vi "运维调试_氨氮.vi"() -> ()   [LabVIEW 2016, in "斯坦道氨氮.lvlib"]
uses:
  <vilib>/Utility/miscctls.llb/LVPointTypeDef.ctl
  <vilib>/Utility/config.llb/NI_LVConfig.lvlib
  <vilib>/ptbypt/NI_PtbyPt.lvlib
panel:
  in  "量程参数读取":T1
  in  "模块启用":bool
  in  "串口设置":bool
  in  "公式一键写入":bool
  in  "流程文件路径":path=path "C:/Users/STD/Documents/斯坦道流程文件/流程.xml"
  in  "曲线模型":cluster{"X^2":dbl, "X":dbl, "B":dbl}(xcontrol)
  in  "质控参数设置":bool
  out "字符串":string
  in  "氨氮自动测试量程配置":T2
  out "ADC":sgl
  out "温度2":sgl
  out "温度1":sgl
  out "固件版本号":string
  in  "数组":string[](array[string])
  in  "备用系数写入":bool
  in  "备用系数读取":bool
  in  "参数下拉列表":enum16{"氨氮", "总磷"}(ring)
  in  "量程下拉列表":enum16{"低量程", "高量程"}(ring)
  in  "测量模式下拉列表":enum16{"水样测量", "空白核查", "跨度核查", "标样核查", "加标回收"}(ring)
  in  "公式":cluster{"X^2":dbl, "X":dbl, "b":dbl}
  in  "写公式":bool
  in  "读公式":bool
  in  "返回":bool
  in  "设置":bool
  out "序列号":string="序列号"
  out "氨氮测量数据":T3(xcontrol)
  out "集成报警信息":string
  out "定时启动":bool
  out "总磷总氮运行状态":T4(xcontrol)
  in  "停止":bool
  in  "手动启动":bool
  in  "单步测试":bool
  in  "总磷氨氮调试":u16[](xcontrol)
  out "F3":sgl format="%#.6f"
  out "F2":sgl format="%#.6f"
  out "F1":sgl format="%#.6f"
  out "F0":sgl format="%#.6f"
  out "多列列表框":i32(listbox)
  # "参数设置"
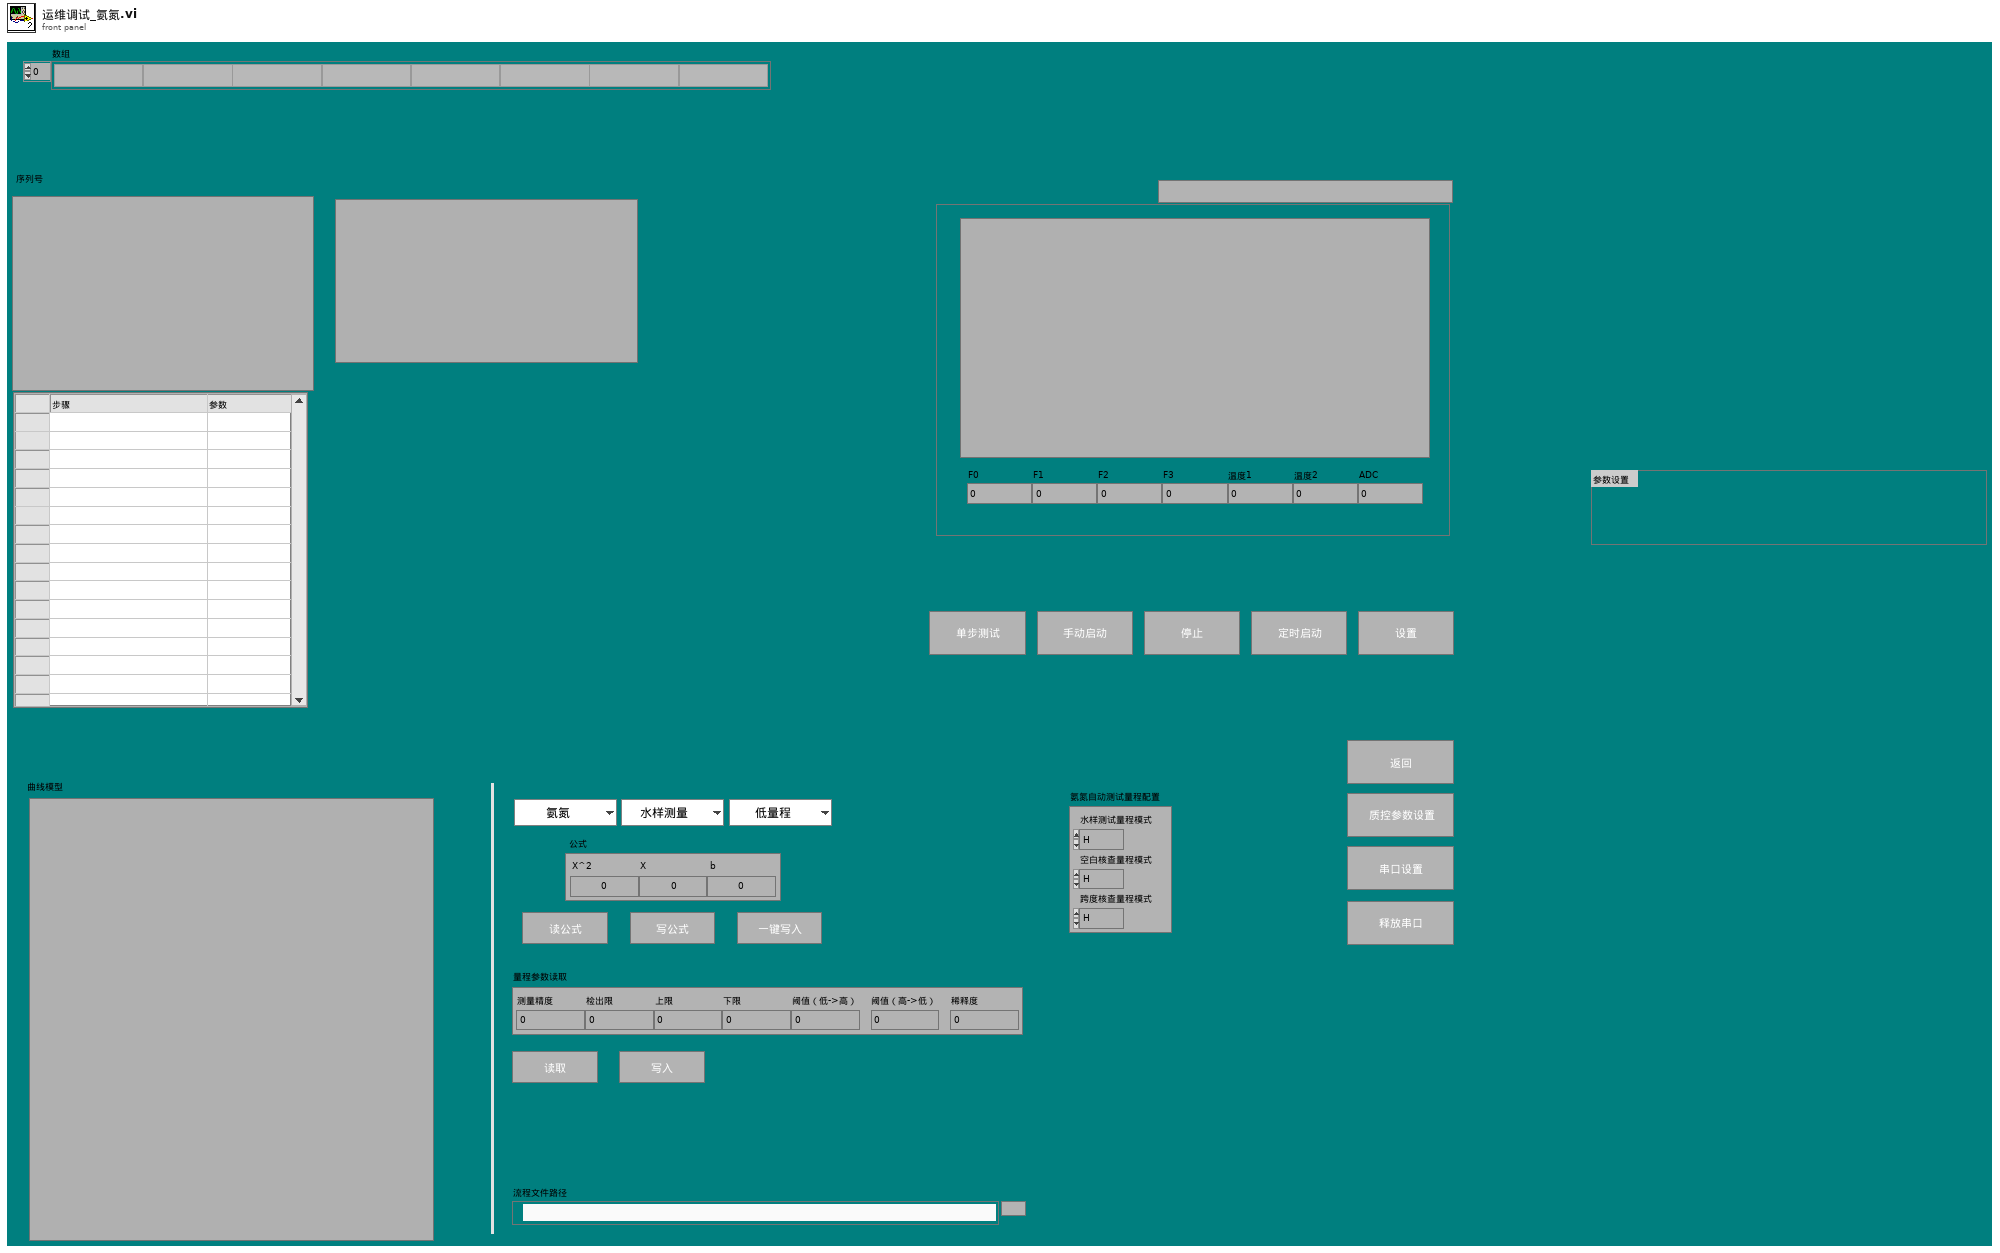
[diagram p1: front panel]
types:
  T1 = cluster{"测量精度":u16, "检出限":dbl, "上限":dbl, "下限":dbl, "阈值（低->高）":dbl, "阈值（高->低）":dbl, "稀释度":dbl}
  T2 = cluster{"水样测试量程模式":enum16{"H", "L", "AUTO"}, "空白核查量程模式":enum16{"H", "L", "AUTO"}, "跨度核查量程模式":enum16{"H", "L", "AUTO"}}
  T3 = cluster{"flowid":u16, "测量精度":u16, "测量数据区":cluster{"因子编码":u32, "单位":u16, "标样参考值":sgl, "水样数据时间":timestamp, "水样实测值":sgl, "水样数据标识":string, "标样数据时间":timestamp, "标样实测值":sgl, "标样数据标识":string, "空白数据时间":timestamp, "空白实测值":sgl, "空白数据标识":string, "零点核查数据时间":timestamp, "零点核查实测值":sgl, "零点核查数据标识":string, "跨度核查数据时间":timestamp, "跨度核查实测值":sgl, "跨度核查数据标识":string, "加标回收数据时间":timestamp, "加标回收实测值":sgl, "加标回收数据标识":string, "平行样数据时间":timestamp, "平行样实测值":sgl, "平行样数据标识":string, "F0":sgl, "F1":sgl, "F2":sgl, "F3":sgl, "F4":sgl, "F5":sgl, "F6":sgl, "F7":sgl, "温度":sgl, "湿度":sgl, "X值":sgl}}
  T4 = cluster{"系统时间":timestamp, "工作状态":enum16{"空闲", "水样测试", "标样核查", "零点核查", "跨度核查", "空白测试", "平行样测试", "加标回收", "空白校准", "标样校准", "初始化（清洗）"}, "测量模式":enum16{"待机", "连续模式", "周期模式", "定点模式", "受控模式", "手动模式"}, "告警代码":enum16{"无告警", "缺试剂告警", "缺水样告警", "缺蒸馏水告警", "缺标液告警", "仪表漏液告警", "标定异常告警", "超量程告警", "加热异常", "低试剂预警", "超上限告警", "超下限告警", "仪表内部其他异常", "滴定异常告警", "电极异常告警", "量程切换告警", "参数设置告警", "PH电极电位异常", "电导率电极异常", "浊度光度异常", "溶解氧电极异常", "溶解氧光强异常", "温度异常告警", "PH异常告警", "溶解氧异常告警", "电导率异常告警", "浊度异常告警", "叶绿素异常告警", "藻密度异常告警", "蓝绿藻异常告警", "ORP异常告警", "氨氮异常告警", "清洁刷异常告警", "SD卡异常告警", "蓝牙异常告警", "Wifi异常告警", "流程异常告警"}, "故障代码":enum16{"无故障", "电机故障", "温度故障", "通讯故障", "滴定故障"}, "日志代码":u16, "软件版本":u16, "F0":sgl, "F1":sgl, "F2":sgl, "F3":sgl, "T":sgl, "H":sgl, "id":u16, "flowid":u16, "量程":u16, "总磷控温温度1":sgl, "营养盐控温温度2":sgl, "ADC":sgl}
  T5 = enum16{"启动测量", "标样核查", "零点核查", "跨度核查", "空白测试", "平行样测试", "加标回收", "空白校准", "标样校准", "初始化（清洗）", "停止测试", "仪器重启", "校时", "模式设置", "测量间隔设置"}
  T6 = cluster{"仪器测试类型":enum16{"启动测量", "标样核查", "零点核查", "跨度核查", "空白测试", "平行样测试", "加标回收", "空白校准", "标样校准", "初始化（清洗）", "停止测试", "仪器重启", "校时", "模式设置", "测量间隔设置"}, "周期设置类型":enum16{"定点启动", "间隔启动"}, "定时功能启用":bool, "定时间隔":dbl, "24H周期设置":bool[], "空白核查时间":u16, "跨度核查时间":u16, "质控频次":enum16{"关闭", "每天", "星期一", "星期二", "星期三", "星期四", "星期五", "星期六", "星期日"}}
  T7 = enum16{"关闭", "每天", "星期一", "星期二", "星期三", "星期四", "星期五", "星期六", "星期日"}
  T8 = enum32{"Bad", "Idle", "Run top level", "Running"}
  T9 = typedef "LVDateTimeRec.ctl" = cluster{"秒数的小数部分":dbl, "秒":i32, "分":i32, "时":i32, "日":i32, "月":i32, "年":i32, "天数（周）":i32, "天数（年）":i32, "DST":i32}
  T10 = typedef "LVPointTypeDef.ctl" = cluster{"Horizontal":i16, "Vertical":i16}
  T11 = cluster{"因子编码":u32, "单位":u16, "标样参考值":sgl, "水样数据时间":timestamp, "水样实测值":sgl, "水样数据标识":string, "标样数据时间":timestamp, "标样实测值":sgl, "标样数据标识":string, "空白数据时间":timestamp, "空白实测值":sgl, "空白数据标识":string, "零点核查数据时间":timestamp, "零点核查实测值":sgl, "零点核查数据标识":string, "跨度核查数据时间":timestamp, "跨度核查实测值":sgl, "跨度核查数据标识":string, "加标回收数据时间":timestamp, "加标回收实测值":sgl, "加标回收数据标识":string, "平行样数据时间":timestamp, "平行样实测值":sgl, "平行样数据标识":string, "F0":sgl, "F1":sgl, "F2":sgl, "F3":sgl, "F4":sgl, "F5":sgl, "F6":sgl, "F7":sgl, "T":sgl, "H":sgl, "X":sgl}
  T12 = enum16{"空闲", "水样测试", "标样核查", "零点核查", "跨度核查", "空白测试", "平行样测试", "加标回收", "空白校准", "标样校准", "初始化（清洗）"}
  T13 = typedef "NI_LVConfig.lvlib/Config Data RefNum.ctl" = refnum<k1>
  T14 = cluster{"启动模式":enum16{"跨度核查", "水样测量", "空白核查", "标样核查", "加标回收"}, "启动参数":u16, "量程":enum16{"低量程", "高量程"}}
  T15 = cluster{"时间标识":timestamp, "设备":string, "日志信息":string, "流程参数":string}
  T16 = cluster{"时间标识":timestamp, "设备":string, "日志信息":string}
  T17 = enum16{"无告警", "缺试剂告警", "缺水样告警", "缺蒸馏水告警", "缺标液告警", "仪表漏液告警", "标定异常告警", "超量程告警", "加热异常", "低试剂预警", "超上限告警", "超下限告警", "仪表内部其他异常", "滴定异常告警", "电极异常告警", "量程切换告警", "参数设置告警", "PH电极电位异常", "电导率电极异常", "浊度光度异常", "溶解氧电极异常", "溶解氧光强异常", "温度异常告警", "PH异常告警", "溶解氧异常告警", "电导率异常告警", "浊度异常告警", "叶绿素异常告警", "藻密度异常告警", "蓝绿藻异常告警", "ORP异常告警", "氨氮异常告警", "清洁刷异常告警", "SD卡异常告警", "蓝牙异常告警", "Wifi异常告警", "流程异常告警"}
  T18 = typedef "LVRowAndColumnUnsignedTypeDef.ctl" = cluster{"Row":u32, "Column":u32}
  T19 = cluster{"站号":u16, "量程切换":enum32{"H", "L", "AUTO"}, "控制命令":enum16{"启动测量", "标样核查", "零点核查", "跨度核查", "空白测试", "平行样测试", "加标回收", "空白校准", "标样校准", "初始化（清洗）", "停止测试", "仪器重启", "校时", "模式设置", "测量间隔设置"}, "模式设置":enum16{"待机", "连续模式", "周期模式", "定点模式", "受控模式", "手动模式"}, "测量间隔":u16}
  T20 = cluster{"跨度值":dbl, "零点标准液浓度":dbl, "跨度标准液浓度":dbl, "标准液标准浓度":dbl}
  T21 = cluster{"确定":bool, "跨度值":dbl, "零点标准液浓度":dbl, "跨度标准液浓度":dbl, "标准液标准浓度":dbl}
  T22 = cluster{"控制命令":enum16{"启动测量", "标样核查", "零点核查", "跨度核查", "空白测试", "平行样测试", "加标回收", "空白校准", "标样校准", "初始化（清洗）", "停止测试", "仪器重启", "校时", "模式设置", "测量间隔设置"}, "周期设置类型":enum16{"定点启动", "间隔启动"}, "定时功能启用":bool, "定时间隔":dbl, "24H周期设置":bool[], "空白核查时间":u16, "跨度核查时间":u16, "质控频次":enum16{"关闭", "每天", "星期一", "星期二", "星期三", "星期四", "星期五", "星期六", "星期日"}}
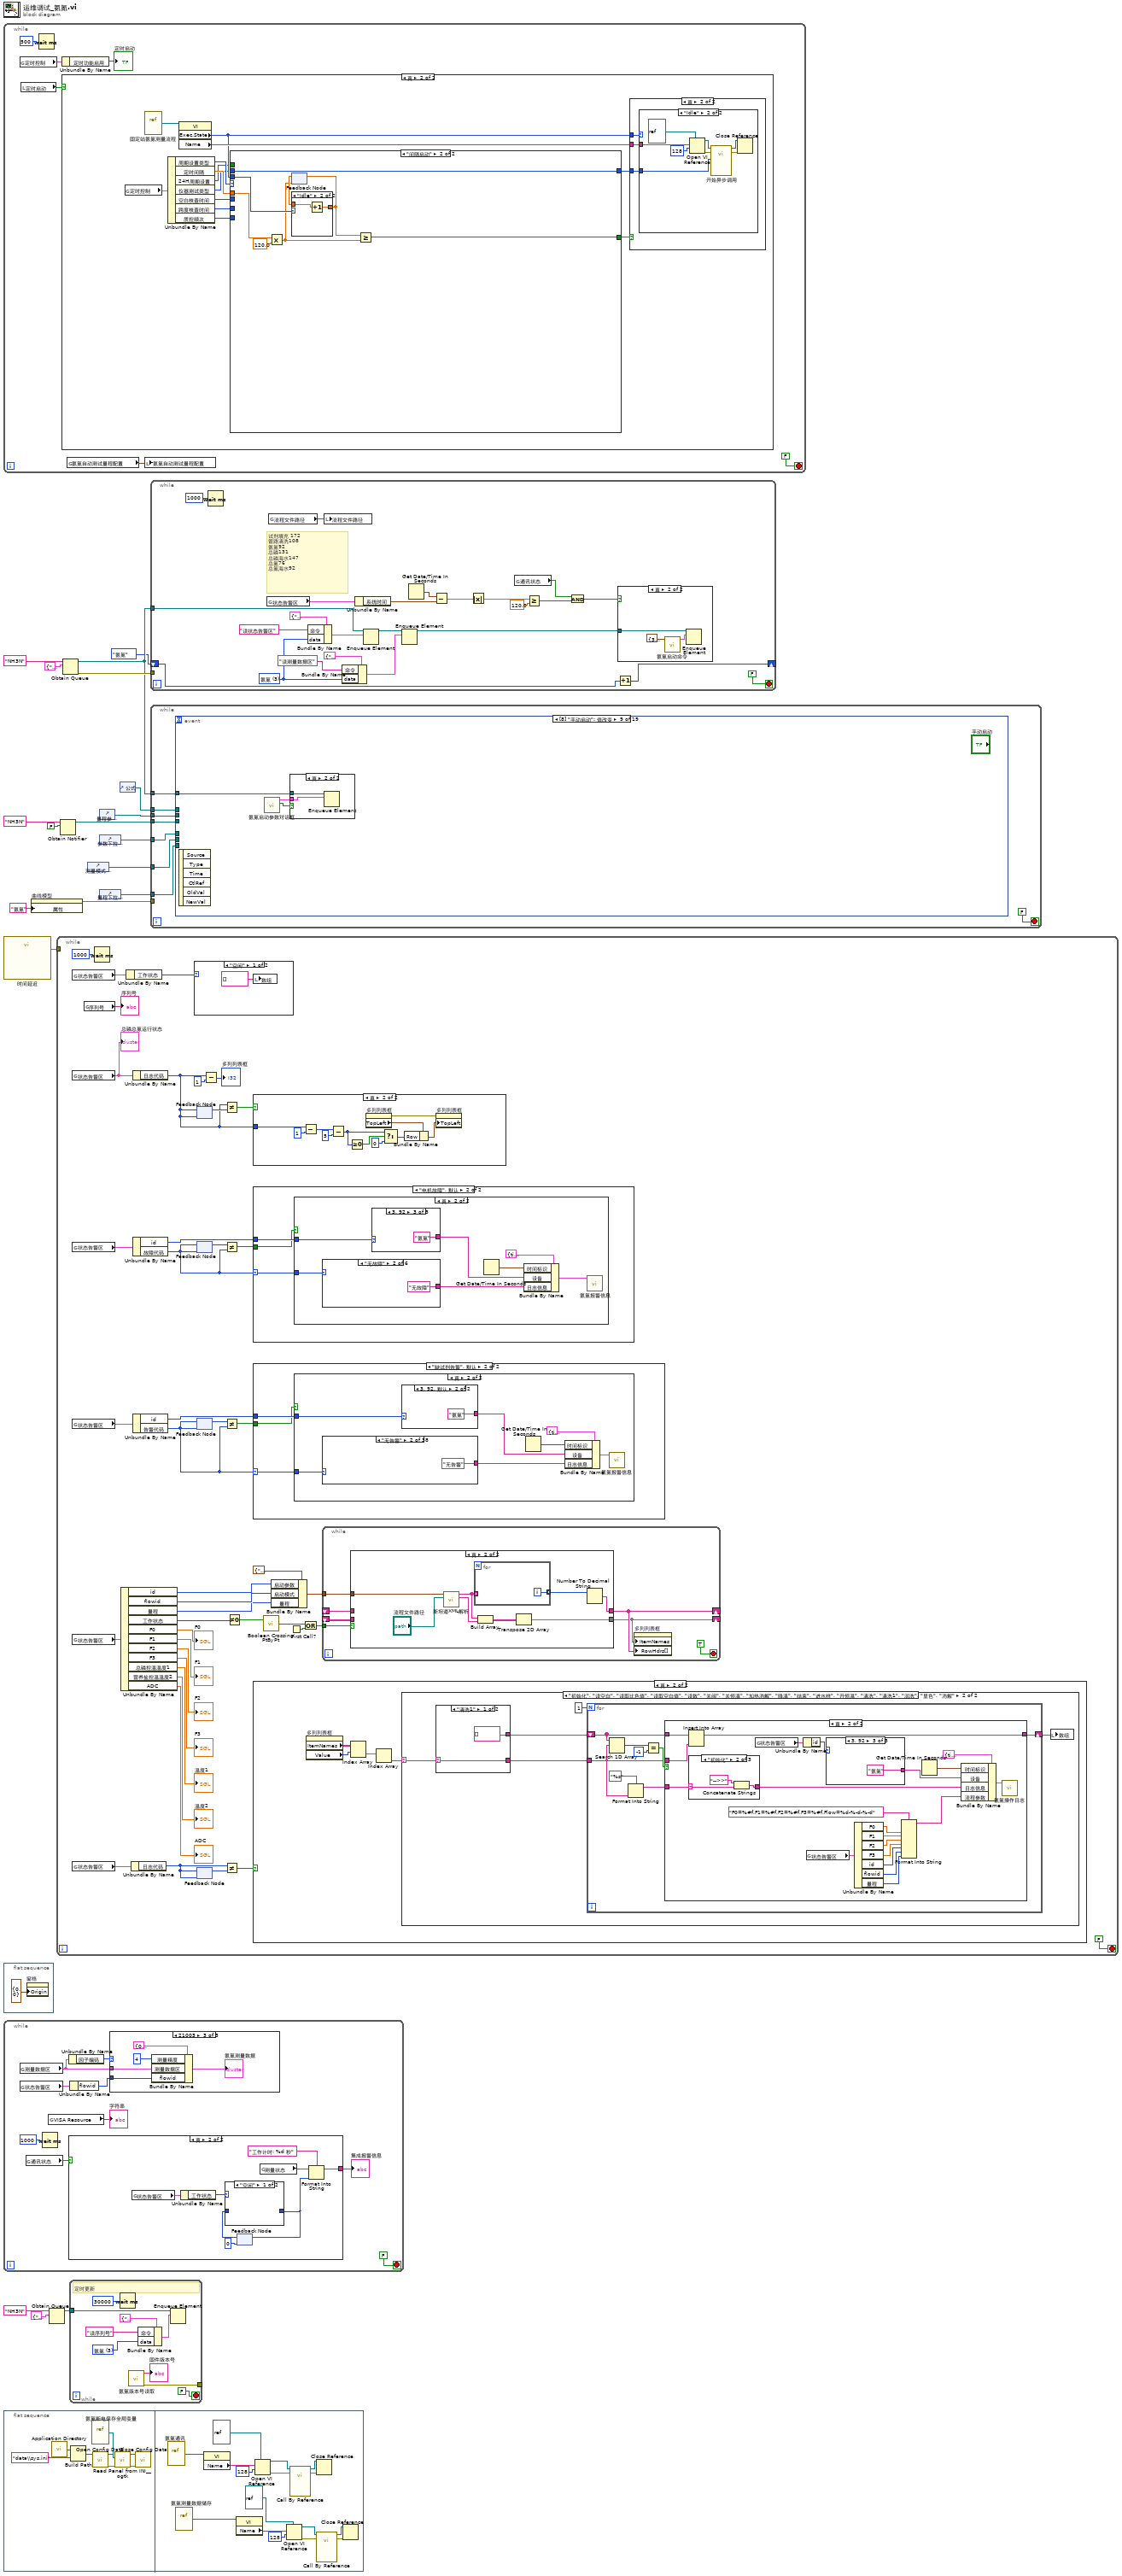
[diagram p0: block diagram]
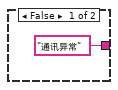
[diagram p2: hidden frame]
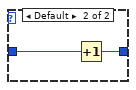
[diagram p3: hidden frame]
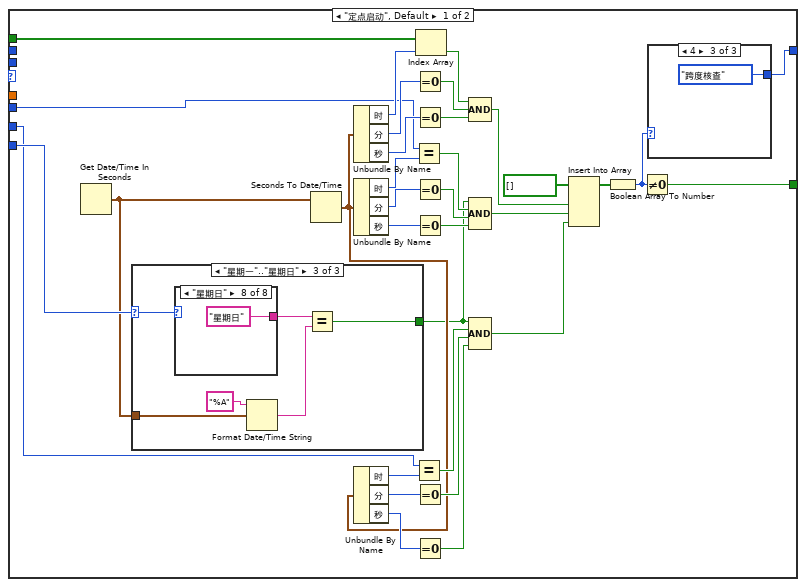
[diagram p7: hidden frame]
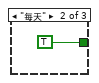
[diagram p9: hidden frame]
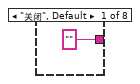
[diagram p10: hidden frame]
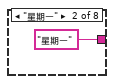
[diagram p11: hidden frame]
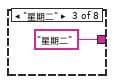
[diagram p12: hidden frame]
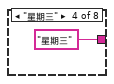
[diagram p13: hidden frame]
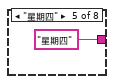
[diagram p14: hidden frame]
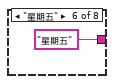
[diagram p15: hidden frame]
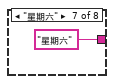
[diagram p16: hidden frame]
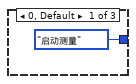
[diagram p17: hidden frame]
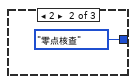
[diagram p18: hidden frame]
diagram:
  n1 = while {
    stop <- FALSE stop-if-true
    n2 = global read "氨氮断电保存全局变量.vi" "定时控制"() -> (w22:T6)
    n3 = local read "定时启动"() -> (w23:bool)
    n4 = Wait (ms)(milliseconds to wait=u32 500 ("等待时间（毫秒）")) -> ()  [unwired: 1 out]
    n5 = Unbundle By Name(w22) -> ("定时功能启用"=→"定时启动":bool)
    n6 = case shown="真" w23 {
      frame False {
      }
      frame True {
        n7 = global read "氨氮断电保存全局变量.vi" "定时控制"() -> (w38:T6)
        n8 = vi-ref "固定站氨氮测量流程.vi"() -> (w37:refnum<vi>)
        n9 = Unbundle By Name(w38) -> ("周期设置类型"=w34:enum16{"定点启动", "间隔启动"}, "定时间隔"=w33:dbl, "24H周期设置"=w32:bool[], "仪器测试类型"=w31:T5, "空白核查时间"=w30:u16, "跨度核查时间"=w29:u16, "质控频次"=w28:T7)
        n10 = property class="VI"(reference=w37) -> ("Exec.State"=w35:T8, "Name"=w36:string)  [unwired: 1 in, 2 out]
        n11 = case shown="\"间隔启动\"" w34 {
          tunnel: w33 -> [_ w94]
          tunnel: w32 -> [w62 _]
          tunnel: w35 -> [_ w97]
          tunnel: [w40 w92] -> w26
          tunnel: w31 -> [_ w90]
          tunnel: [w66 w90] -> w27
          tunnel: w28 -> [w65 _]
          tunnel: w30 -> [w58 _]
          tunnel: w29 -> [w47 _]
          frame "定点启动", Default {
            n12 = Get Date/Time In Seconds() -> (seconds since 1Jan1904=w64:timestamp)
            n13 = case shown="\"星期一\"..\"星期日\"" w65 {
              selector: w65 -> [_ _ w76]
              tunnel: w64 -> [_ _ w77]
              tunnel: [_ TRUE w73] -> w46
              frame "关闭", Default {
              }
              frame "每天" {
              }
              frame "星期一".."星期日" {
                n14 = case shown="\"星期日\"" w76 {
                  tunnel: ["" ("时间格式字符串(%c)") "星期一" ("时间格式字符串(%c)") "星期二" ("时间格式字符串(%c)") "星期三" ("时间格式字符串(%c)") "星期四" ("时间格式字符串(%c)") "星期五" ("时间格式字符串(%c)") "星期六" ("时间格式字符串(%c)") "星期日" ("时间格式字符串(%c)")] -> w75
                  frame "关闭", Default {
                  }
                  frame "星期一" {
                  }
                  frame "星期二" {
                  }
                  frame "星期三" {
                  }
                  frame "星期四" {
                  }
                  frame "星期五" {
                  }
                  frame "星期六" {
                  }
                  frame "星期日" {
                  }
                }
                n15 = Format Date/Time String(time format string (%c)="%A" ("时间格式字符串(%c)"), seconds (now)=w77) -> (date/time string=w74:string)  [unwired: 1 in]
                n16 = Equal?(x=w75, y=w74) -> (x = y?=w73:bool)
              }
            }
            n17 = Seconds To Date/Time(time stamp (now)=w64) -> (date time rec=w48:T9)  [unwired: 1 in]
            n18 = Unbundle By Name(w48) -> ("时"=w71:i32, "分"=w69:i32, "秒"=w70:i32)
            n19 = Unbundle By Name(w48) -> ("时"=w59:i32, "分"=w61:i32, "秒"=w60:i32)
            n20 = Unbundle By Name(w48) -> ("时"=w51:i32, "分"=w49:i32, "秒"=w50:i32)
            n21 = Equal?(x=w58, y=w59) -> (x = y?=w57:bool)
            n22 = Equal?(x=w47, y=w51) -> (x = y?=w52:bool)
            n23 = Equal To 0?(x=w69) -> (x = 0?=w68:bool)
            n24 = Equal To 0?(x=w70) -> (x = 0?=w67:bool)
            n25 = Equal To 0?(x=w61) -> (x = 0?=w56:bool)
            n26 = Equal To 0?(x=w60) -> (x = 0?=w55:bool)
            n27 = Equal To 0?(x=w49) -> (x = 0?=w53:bool)
            n28 = Equal To 0?(x=w50) -> (x = 0?=w54:bool)
            n29 = Index Array(array=w62, index=w71) -> (element=w63:bool)
            n30 = Compound Arithmetic op=AND ("复合运算")(w63, w68, w67) -> (w44:bool)
            n31 = Compound Arithmetic op=AND ("复合运算")(w46, w57, w56, w55) -> (w43:bool)
            n32 = Compound Arithmetic op=AND ("复合运算")(w46, w52, w53, w54) -> (w42:bool)
            n33 = Insert Into Array(array=bool[] [], new element #1=w44, new element #2=w43, new element #3=w42) -> (w41:bool[])  [unwired: 1 in]
            n34 = Boolean Array To Number(Boolean array=w41) -> (number=w39:u32)
            n35 = Not Equal To 0?(x=w39) -> (x != 0?=w40:bool)
            n36 = case shown="4" w39 {
              tunnel: [T5."启动测量" ("控制命令") T5."零点核查" ("控制命令") T5."跨度核查" ("控制命令")] -> w66
              frame 0, Default {
              }
              frame 2 {
              }
              frame 4 {
              }
            }
          }
          frame "间隔启动" {
            n37 = Multiply(x=w94, y=120.0) -> (x*y=w91:dbl)
            n38 = feedback #1(w91) -> (w96:dbl)
            n39 = case shown="\"Idle\"" w97 {
              tunnel: w96 -> [_ w99]
              tunnel: [_ w98] -> w95
              frame "Bad", Default {
              }
              frame "Idle" {
                n40 = Increment(x=w99) -> (x+1=w98:dbl)
              }
            }
            n41 = feedback-in #1(w95) -> ()
            n42 = Greater Or Equal?(x=w95, y=w91) -> (x >= y?=w92:bool)
          }
        }
        n43 = case shown="真" w26 {
          tunnel: w36 -> [_ w102]
          tunnel: w27 -> [_ w101]
          tunnel: w35 -> [_ w100]
          frame False {
          }
          frame True {
            n44 = case shown="\"Idle\"" w100 {
              tunnel: w102 -> [_ w106]
              tunnel: w101 -> [_ w103]
              frame "Bad", Default {
              }
              frame "Idle" {
                n45 = Open VI Reference(type specifier VI Refnum (for type only)=refnum<vi> refnum, vi path=w106, options=128 ("选项")) -> (vi reference=w107:refnum<vi>, error out=w108:errorcluster)  [unwired: 3 in]
                n46 = call-by-ref "开始异步调用"(reference=w107, error in=w108, "控制命令"=w103) -> (reference out=w109:refnum<vi>, error out=w110:errorcluster)  [unwired: 11 in]
                n47 = Close Reference(reference=w109, error in (no error)=w110) -> ()  [unwired: 1 out]
              }
            }
          }
        }
      }
    }
    n48 = global read "氨氮断电保存全局变量.vi" "氨氮自动测试量程配置"() -> (w20:T2)
    n49 = local write "氨氮自动测试量程配置"(w20) -> ()
  }
  n50 = call "时间延迟"() -> ("error out"=w10:errorcluster)  [unwired: 11 in]
  n51 = flat-sequence {
    frame #0 {
      n52 = property on="窗格" class="Pane"("Origin"=T10 {"Horizontal"=0, "Vertical"=0} ("原点")) -> ()  [unwired: 2 in, 2 out]
    }
  }
  n53 = while {
    stop <- FALSE stop-if-true
    n54 = global read "VAR氨氮全局变量.vi" "测量数据区"() -> (w118:T11)
    n55 = global read "VAR氨氮全局变量.vi" "状态告警区"() -> (w114:T4)
    n56 = global read "VAR氨氮全局变量.vi" "通讯状态"() -> (w116:bool)
    n57 = Wait (ms)(milliseconds to wait=u32 1000 ("等待时间（毫秒）")) -> ()  [unwired: 1 out]
    n58 = global read "氨氮断电保存全局变量.vi" "VISA Resource"() -> (→"字符串":refnum<visa-resource-name>)
    n59 = Unbundle By Name(w118) -> ("因子编码"=w117:u32)
    n60 = case shown="真" w116 {
      tunnel: ["通讯异常" ("集成报警信息") w123] -> w115
      frame False {
      }
      frame True {
        n61 = global read "VAR氨氮全局变量.vi" "状态告警区"() -> (w129:T4)
        n62 = Unbundle By Name(w129) -> ("工作状态"=w128:T12)
        n63 = feedback #2(0) -> (w126:i32)
        n64 = case shown="\"空闲\"" w128 {
          tunnel: w126 -> [_ w131]
          tunnel: [_ w130] -> w124
          frame "空闲" {
          }
          frame Default {
            n65 = Increment(x=w131) -> (x+1=w130:i32)
          }
        }
        n66 = feedback-in #2(w124) -> ()
        n67 = global read "VAR氨氮全局变量.vi" "测量状态"() -> (w122:string)
        n68 = Format Into String(format string="工作计时: %d 秒" ("格式字符串"), initial string=w122, w124) -> (resulting string=w123:string)  [unwired: 1 in, 1 out]
      }
    }
    "集成报警信息" <- w115
    n69 = Unbundle By Name(w114) -> ("flowid"=w113:u16)
    n70 = case shown="21003" w117 {
      tunnel: w118 -> [_ _ w136]
      tunnel: w113 -> [_ _ w134]
      frame Default {
      }
      frame 21011 {
      }
      frame 21003 {
        n71 = Bundle By Name(cluster=T3 {"flowid"=0, "测量精度"=0, "测量数据区"={"因子编码"=0, "单位"=0, "标样参考值"=0.0, "水样数据时间"=timestamp(0 s since 1904-01-01), "水样实测值"=0.0, "水样数据标识"="", "标样数据时间"=timestamp(0 s since 1904-01-01), "标样实测值"=0.0, "标样数据标识"="", "空白数据时间"=timestamp(0 s since 1904-01-01), "空白实测值"=0.0, "空白数据标识"="", "零点核查数据时间"=timestamp(0 s since 1904-01-01), "零点核查实测值"=0.0, "零点核查数据标识"="", "跨度核查数据时间"=timestamp(0 s since 1904-01-01), "跨度核查实测值"=0.0, "跨度核查数据标识"="", "加标回收数据时间"=timestamp(0 s since 1904-01-01), "加标回收实测值"=0.0, "加标回收数据标识"="", "平行样数据时间"=timestamp(0 s since 1904-01-01), "平行样实测值"=0.0, "平行样数据标识"="", "F0"=0.0, "F1"=0.0, "F2"=0.0, "F3"=0.0, "F4"=0.0, "F5"=0.0, "F6"=0.0, "F7"=0.0, "温度"=0.0, "湿度"=0.0, "X值"=0.0}} ("氨氮测量数据"), "测量精度"=u16 4, "测量数据区"=w136, "flowid"=w134) -> (→"氨氮测量数据":T3)
      }
    }
  }
  n72 = flat-sequence {
    frame #0 {
      n73 = call <vilib>:"Application Directory.vi"() -> ("Application Directory"=w137:path)
      n74 = Build Path(base path=w137, name or relative path="data\\sys.ini" ("名称或相对路径")) -> (appended path=w139:path)
      n75 = vi-ref "氨氮断电保存全局变量.vi"() -> (w141:refnum<vi>)
      n76 = call <vilib>:"Open Config Data.vi"("configuration file path"=w139) -> ("error out"=w143:errorcluster, "refnum"=w140:T13)  [unwired: 8 in, 1 out]
      n77 = call <userlib>:"Read Panel from INI__ogtk.vi"("error in (no error)"=w143, "VI ref"=w141, "refnum"=w140) -> ("error out"=w144:errorcluster, "refnum out"=w142:T13)  [unwired: 7 in]
      n78 = call <vilib>:"Close Config Data.vi"("error in (no error)"=w144, "refnum"=w142) -> ()  [unwired: 8 in, 2 out]
    }
    frame #1 {
      n79 = vi-ref "氨氮通讯.vi"() -> (w160:refnum<vi>)
      n80 = vi-ref "氨氮测量数据储存.vi"() -> (w152:refnum<vi>)
      n81 = property class="VI"(reference=w160) -> ("Name"=w159:string)  [unwired: 1 in, 2 out]
      n82 = property class="VI"(reference=w152) -> ("Name"=w145:string)  [unwired: 1 in, 2 out]
      n83 = Open VI Reference(type specifier VI Refnum (for type only)=refnum<vi> refnum, vi path=w159, options=128 ("选项")) -> (vi reference=w157:refnum<vi>, error out=w155:errorcluster)  [unwired: 3 in]
      n84 = Open VI Reference(type specifier VI Refnum (for type only)=refnum<vi> refnum, vi path=w145, options=128 ("选项")) -> (vi reference=w147:refnum<vi>, error out=w149:errorcluster)  [unwired: 3 in]
      n85 = call-by-ref "?"(reference=w157, error in=w155) -> (reference out=w153:refnum<vi>, error out=w154:errorcluster)  [unwired: 12 in]
      n86 = Close Reference(reference=w153, error in (no error)=w154) -> ()  [unwired: 1 out]
      n87 = call-by-ref "?"(reference=w147, error in=w149) -> (reference out=w151:refnum<vi>, error out=w150:errorcluster)  [unwired: 12 in]
      n88 = Close Reference(reference=w151, error in (no error)=w150) -> ()  [unwired: 1 out]
    }
  }
  n89 = property on="曲线模型" class="曲线模型 (严格)"("属性"="氨氮" ("调用模块名称属性")) -> (error out=w3:errorcluster)  [unwired: 2 in, 1 out]
  n90 = Obtain Queue(name (unnamed)="NH3N" ("名称（未命名）"), element data type=cluster{"命令":string, "data":variant} {"命令"="", "data"=variant}) -> (queue out=w7:refnum<queue>)  [unwired: 3 in, 2 out]
  n91 = while {
    tunnel: w10 -> [_]
    stop <- FALSE stop-if-true
    n92 = global read "VAR氨氮全局变量.vi" "状态告警区"() -> (w176:T4)
    n93 = global read "VAR氨氮全局变量.vi" "状态告警区"() -> (w188:T4)
    "总磷总氮运行状态" <- w188
    n94 = global read "VAR氨氮全局变量.vi" "状态告警区"() -> (w181:T4)
    n95 = global read "VAR氨氮全局变量.vi" "状态告警区"() -> (w186:T4)
    n96 = global read "VAR氨氮全局变量.vi" "状态告警区"() -> (w196:T4)
    n97 = global read "VAR氨氮全局变量.vi" "状态告警区"() -> (w173:T4)
    n98 = global read "VAR氨氮全局变量.vi" "序列号"() -> (→"序列号":string)
    n99 = Wait (ms)(milliseconds to wait=u32 1000 ("等待时间（毫秒）")) -> ()  [unwired: 1 out]
    n100 = Unbundle By Name(w196) -> ("id"=w193:u16, "flowid"=w195:u16, "量程"=w194:u16, "工作状态"=w162:T12, "F0"=→"F0":sgl, "F1"=→"F1":sgl, "F2"=→"F2":sgl, "F3"=→"F3":sgl, "总磷控温温度1"=→"温度1":sgl, "营养盐控温温度2"=→"温度2":sgl, "ADC"=→"ADC":sgl)
    n101 = Unbundle By Name(w176) -> ("工作状态"=w175:T12)
    n102 = Unbundle By Name(w173) -> ("日志代码"=w172:u16)
    n103 = Unbundle By Name(w188) -> ("日志代码"=w166:u16)
    n104 = Unbundle By Name(w181) -> ("id"=w180:u16, "故障代码"=w177:enum16{"无故障", "电机故障", "温度故障", "通讯故障", "滴定故障"})
    n105 = Unbundle By Name(w186) -> ("id"=w185:u16, "告警代码"=w182:T17)
    n106 = case shown="\"空闲\"" w175 {
      frame "空闲" {
        n107 = local write "数组"(string[] [] ("数组")) -> ()
      }
      frame "水样测试", Default {
      }
    }
    n108 = feedback-in #3(w166) -> ()
    n109 = feedback #3(w166) -> (w201:u16)
    n110 = feedback #4(w177) -> (w178:enum16{"无故障", "电机故障", "温度故障", "通讯故障", "滴定故障"})
    n111 = feedback-in #4(w177) -> ()
    n112 = feedback #5(w182) -> (w183:T17)
    n113 = feedback-in #5(w182) -> ()
    n114 = feedback #6(w172) -> (w174:u16)
    n115 = feedback-in #6(w172) -> ()
    n116 = Subtract(x=w166, y=1) -> (x-y=→"多列列表框":i32)
    n117 = Not Equal?(x=w166, y=w201) -> (x != y?=w200:bool)
    n118 = Not Equal?(x=w178, y=w177) -> (x != y?=w179:bool)
    n119 = Not Equal?(x=w183, y=w182) -> (x != y?=w184:bool)
    n120 = Not Equal?(x=w172, y=w174) -> (x != y?=w171:bool)
    n121 = Not Equal To 0?(x=w162) -> (x != 0?=w198:bool)
    n122 = case shown="真" w200 {
      tunnel: w166 -> [_ w351]
      frame False {
      }
      frame True {
        n123 = Subtract(x=w351, y=1) -> (x-y=w349:i32)
        n124 = Subtract(x=w349, y=5) -> (x-y=w353:i32)
        n125 = Greater Or Equal To 0?(x=w353) -> (x >= 0?=w352:bool)
        n126 = property on="多列列表框" class="MCListbox (严格)"() -> (error out=w357:errorcluster, "TopLeft"=w358:T18)  [unwired: 2 in, 1 out]
        n127 = Select(t=w353, s=w352, f=0) -> (s? t:f=w354:i32)
        n128 = Bundle By Name(cluster=w358, "Row"=w354) -> (w359:T18)
        n129 = property on="多列列表框" class="MCListbox (严格)"(error in=w357, "TopLeft"=w359) -> ()  [unwired: 1 in, 2 out]
      }
    }
    n130 = case shown="\"电机故障\", 默认" w177 {
      selector: w177 -> [_ w258]
      tunnel: w180 -> [_ w259]
      tunnel: w179 -> [_ w257]
      frame "无故障" {
      }
      frame "电机故障", Default {
        n131 = case shown="真" w257 {
          tunnel: w259 -> [_ w266]
          tunnel: w258 -> [_ w261]
          frame False {
          }
          frame True {
            n132 = case shown="\"无故障\"" w261 {
              selector: w261 -> [w268 _ _ _ _ _]
              tunnel: [w267 "无故障" "电机故障" "温度故障" "通讯故障" "滴定故障"] -> w260
              frame Default {
                n133 = Format Into String(format string="%d" ("格式字符串"), initial string="未知" ("工作状态"), w268) -> (resulting string=w267:string)  [unwired: 1 in, 1 out]
              }
              frame "无故障" {
              }
              frame "电机故障" {
              }
              frame "温度故障" {
              }
              frame "通讯故障" {
              }
              frame "滴定故障" {
              }
            }
            n134 = case shown="3, 92" w266 {
              tunnel: [_ "总磷" ("table输入") "氨氮" ("table输入")] -> w262
              frame Default {
              }
              frame 1, 131 {
              }
              frame 3, 92 {
              }
            }
            n135 = Get Date/Time In Seconds() -> (seconds since 1Jan1904=w263:timestamp)
            n136 = Bundle By Name(cluster=T16 {"时间标识"=timestamp(0 s since 1904-01-01), "设备"="", "日志信息"=""} ("data in"), "时间标识"=w263, "设备"=w262, "日志信息"=w260) -> (w264:T16)
            n137 = call "氨氮报警信息.vi"("data in"=w264) -> ()  [unwired: 10 in, 1 out]
          }
        }
      }
    }
    n138 = case shown="\"缺试剂告警\", 默认" w182 {
      selector: w182 -> [_ w279]
      tunnel: w185 -> [_ w280]
      tunnel: w184 -> [_ w278]
      frame "无告警" {
      }
      frame "缺试剂告警", Default {
        n139 = case shown="真" w278 {
          tunnel: w280 -> [_ w287]
          tunnel: w279 -> [_ w281]
          frame False {
          }
          frame True {
            n140 = case shown="\"无告警\"" w281 {
              selector: w281 -> [w289 _ _ _ _ _ _ _ _ _ _ _ _ _ _ _ _ _ _ _ _ _ _ _ _ _ _ _ _ _ _ _ _ _ _ _ _ _]
              tunnel: [w288 "无告警" "缺试剂告警" "缺水样告警" "缺蒸馏水告警" "缺标液告警" "仪表漏液告警" "标定异常告警" "超量程告警" "加热异常" "低试剂预警" "超上限告警" "超下限告警" "仪表内部其他异常" "滴定异常告警" "电极异常告警" "量程切换告警" "参数设置告警" "PH电极电位异常" "电导率电极异常" "浊度光度异常" "溶解氧电极异常" "溶解氧光强异常" "温度异常告警" "PH异常告警" "溶解氧异常告警" "电导率异常告警" "浊度异常告警" "叶绿素异常告警" "藻密度异常告警" "蓝绿藻异常告警" "ORP异常告警" "氨氮异常告警" "清洁刷异常告警" "SD卡异常告警" "蓝牙异常告警" "WiFi异常告警" "流程异常告警"] -> w282
              frame Default {
                n141 = Format Into String(format string="%d" ("格式字符串"), initial string="未知" ("工作状态"), w289) -> (resulting string=w288:string)  [unwired: 1 in, 1 out]
              }
              frame "无告警" {
              }
              frame "缺试剂告警" {
              }
              frame "缺水样告警" {
              }
              frame "缺蒸馏水告警" {
              }
              frame "缺标液告警" {
              }
              frame "仪表漏液告警" {
              }
              frame "标定异常告警" {
              }
              frame "超量程告警" {
              }
              frame "加热异常" {
              }
              frame "低试剂预警" {
              }
              frame "超上限告警" {
              }
              frame "超下限告警" {
              }
              frame "仪表内部其他异常" {
              }
              frame "滴定异常告警" {
              }
              frame "电极异常告警" {
              }
              frame "量程切换告警" {
              }
              frame "参数设置告警" {
              }
              frame "PH电极电位异常" {
              }
              frame "电导率电极异常" {
              }
              frame "浊度光度异常" {
              }
              frame "溶解氧电极异常" {
              }
              frame "溶解氧光强异常" {
              }
              frame "温度异常告警" {
              }
              frame "PH异常告警" {
              }
              frame "溶解氧异常告警" {
              }
              frame "电导率异常告警" {
              }
              frame "浊度异常告警" {
              }
              frame "叶绿素异常告警" {
              }
              frame "藻密度异常告警" {
              }
              frame "蓝绿藻异常告警" {
              }
              frame "ORP异常告警" {
              }
              frame "氨氮异常告警" {
              }
              frame "清洁刷异常告警" {
              }
              frame "SD卡异常告警" {
              }
              frame "蓝牙异常告警" {
              }
              frame "Wifi异常告警" {
              }
              frame "流程异常告警" {
              }
            }
            n142 = case shown="3, 92, 默认" w287 {
              tunnel: ["总磷" ("table输入") "氨氮" ("table输入")] -> w283
              frame 1, 131 {
              }
              frame 3, 92, Default {
              }
            }
            n143 = Get Date/Time In Seconds() -> (seconds since 1Jan1904=w284:timestamp)
            n144 = Bundle By Name(cluster=T16 {"时间标识"=timestamp(0 s since 1904-01-01), "设备"="", "日志信息"=""} ("data in"), "时间标识"=w284, "设备"=w283, "日志信息"=w282) -> (w285:T16)
            n145 = call "氨氮报警信息.vi"("data in"=w285) -> ()  [unwired: 10 in, 1 out]
          }
        }
      }
    }
    n146 = case shown="真" w171 {
      frame False {
      }
      frame True {
        n147 = property on="多列列表框" class="MCListbox (严格)"() -> ("ItemNames"=w207:string[][], "Value"=w208:i32)  [unwired: 2 in, 2 out]
        n148 = Index Array(array=w207, index (row)=w208) -> (element=w206:string[])  [unwired: 1 in]
        n149 = Index Array(array=w206) -> (element=w205:string)  [unwired: 1 in]
        n150 = case shown="\"初始化\", \"读空白\", \"读取比色值\", \"读取空白值\", \"读数\", \"关阀\", \"关恒温\", \"加热消解\", \"降温\", \"结束\", \"进水样\", \"开恒温\", \"清洗\", \"清洗1\", \"润洗\", \"显色\", \"消解\"" w205 {
          selector: w205 -> [_ w211]
          frame Default {
          }
          frame "初始化", "读空白", "读取比色值", "读取空白值", "读数", "关阀", "关恒温", "加热消解", "降温", "结束", "进水样", "开恒温", "清洗", "清洗1", "润洗", "显色", "消解" {
            n151 = case shown="\"清洗1\"" w211 {
              selector: w211 -> [w215 w217]
              tunnel: [w215 w217] -> w210
              tunnel: [string[] [] ("数组") "数组"] -> w209
              frame "清洗1" {
              }
              frame Default {
              }
            }
            n152 = for {
              N: 1 -> [_]
              tunnel: w210 -> [w219]
              shift-right: [w218] -> w212
              shift-left: w209 -> [w220]
              n153 = Search 1D Array(1D array=w220, element=w219) -> (index of element=w223:i32)  [unwired: 1 in]
              n154 = Format Into String(format string="%s" ("格式字符串"), w219) -> (resulting string=w224:string)  [unwired: 2 in, 1 out]
              n155 = Equal?(x=w223, y=-1) -> (x = y?=w221:bool)
              n156 = case shown="真" w221 {
                tunnel: w224 -> [_ w228]
                tunnel: w220 -> [w226 w232]
                tunnel: w219 -> [_ w231]
                tunnel: [w226 w230] -> w218
                frame False {
                }
                frame True {
                  n157 = Insert Into Array(array=w232, new element=w231) -> (w230:string[])  [unwired: 1 in]
                  n158 = case shown="\"初始化\"" w228 {
                    selector: w228 -> [w248 w251 w254]
                    tunnel: [w248 w250 w253] -> w227
                    frame Default {
                    }
                    frame "初始化" {
                      n159 = Concatenate Strings("-->>" ("字符串"), w251) -> (w250:string)
                    }
                    frame "结束" {
                      n160 = Concatenate Strings("-->>" ("字符串"), w254) -> (w253:string)
                    }
                  }
                  n161 = global read "VAR氨氮全局变量.vi" "状态告警区"() -> (w247:T4)
                  n162 = Unbundle By Name(w247) -> ("id"=w246:u16)
                  n163 = global read "VAR氨氮全局变量.vi" "状态告警区"() -> (w242:T4)
                  n164 = case shown="3, 92" w246 {
                    tunnel: [_ "总磷" ("table输入") "氨氮" ("table输入")] -> w244
                    frame Default {
                    }
                    frame 1, 131 {
                    }
                    frame 3, 92 {
                    }
                  }
                  n165 = Unbundle By Name(w242) -> ("F0"=w239:sgl, "F1"=w238:sgl, "F2"=w237:sgl, "F3"=w236:sgl, "id"=w235:u16, "flowid"=w234:u16, "量程"=w233:u16)
                  n166 = Format Into String(format string="F0=%#f,F1=%#f,F2=%#f,F3=%#f,Flow=%d-%-d-%-d" ("格式字符串"), w239, w238, w237, w236, w235, w234, w233) -> (resulting string=w240:string)  [unwired: 2 in, 1 out]
                  n167 = Get Date/Time In Seconds() -> (seconds since 1Jan1904=w243:timestamp)
                  n168 = Bundle By Name(cluster=T15 {"时间标识"=timestamp(0 s since 1904-01-01), "设备"="", "日志信息"="", "流程参数"=""} ("data in"), "时间标识"=w243, "设备"=w244, "日志信息"=w227, "流程参数"=w240) -> (w245:T15)
                  n169 = call "氨氮操作日志.vi"("data in"=w245) -> ()  [unwired: 11 in]
                }
              }
            }
            n170 = local write "数组"(w212) -> ()
          }
        }
      }
    }
    n171 = call <vilib>:"Boolean Crossing PtByPt.vi"("input"=w198) -> ("crossing"=w161:bool)  [unwired: 2 in]
    n172 = Bundle By Name(cluster=T14 {"启动模式"=enum."跨度核查", "启动参数"=1, "量程"=enum."低量程"} ("参数簇"), "启动参数"=w193, "启动模式"=w195, "量程"=w194) -> (w163:T14)
    n173 = First Call?() -> (First Call?: T/F=w199:bool)
    n174 = Or(x=w161, y=w199) -> (x .or. y?=w197:bool)
    n175 = while {
      tunnel: w197 -> [w337]
      tunnel: w163 -> [w336]
      shift-right: [w331] -> _
      shift-left: _ -> [w333]
      shift-right: [w332] -> _
      shift-left: _ -> [w334]
      stop <- TRUE stop-if-true
      n176 = case shown="真" w337 {
        tunnel: [w339 w347] -> w332
        tunnel: [w338 w346] -> w331
        tunnel: w336 -> [_ w341]
        tunnel: w334 -> [w339 _]
        tunnel: w333 -> [w338 _]
        frame False {
        }
        frame True {
          n177 = call "斯坦道XML解析.vi"("添加的路径"="流程文件路径", "参数簇"=w341) -> ("步骤时间"=w342:string[], "步骤名"=w344:string[])  [unwired: 8 in]
          n178 = for {
            tunnel: w344 -> [_] mode=indexing
            tunnel: [w348] -> w345 mode=indexing
            i -> [w348]
          }
          n179 = Build Array(w344, w342) -> (w343:string[][])
          n180 = Transpose 2D Array(2D array=w343) -> (transposed array=w346:string[][])
          n181 = Number To Decimal String(number=w345) -> (decimal integer string=w347:string[])  [unwired: 1 in]
        }
      }
      n182 = property on="多列列表框" class="MCListbox (严格)"("ItemNames"=w331, "RowHdrs[]"=w332) -> ()  [unwired: 2 in, 2 out]
    }
  }
  n183 = Obtain Notifier(name (unnamed)="NH3N" ("名称（未命名）"), notification data type=FALSE) -> (notifier out=w4:refnum<notifier>)  [unwired: 2 in, 2 out]
  n184 = Obtain Queue(name (unnamed)="NH3N" ("名称（未命名）"), element data type=cluster{"命令":string, "data":variant} {"命令"="", "data"=variant}) -> (queue out=w16:refnum<queue>, error out=w17:errorcluster)  [unwired: 3 in, 1 out]
  n185 = while {
    tunnel: w7 -> [w364]
    tunnel: [w361] -> _
    stop <- FALSE stop-if-true
    w365 = u16 3 items=["总磷"=1, "氨氮"=3] ("站号")
    # "定时更新"
    n186 = Wait (ms)(milliseconds to wait=u32 30000 ("等待时间（毫秒）")) -> ()  [unwired: 1 out]
    n187 = call "氨氮版本号读取.vi"() -> ("error out"=w361:errorcluster, "固件版本号"=→"固件版本号":string)  [unwired: 10 in]
    n188 = Bundle By Name(cluster=cluster{"命令":string, "data":variant} {"命令"="", "data"=variant} ("元素"), "命令"="读序列号", "data"=w365) -> (w363:cluster{"命令":string, "data":variant})
    n189 = Enqueue Element(queue=w364, element=w363) -> ()  [unwired: 2 in, 3 out]
  }
  n190 = control-ref of="测量模式下拉列表"() -> (w12:refnum<vi>)
  n191 = control-ref of="量程参数读取"() -> (w1:refnum<vi>)
  n192 = control-ref of="参数下拉列表"() -> (w13:refnum<vi>)
  n193 = control-ref of="量程下拉列表"() -> (w14:refnum<vi>)
  n194 = control-ref of="公式"() -> (w11:refnum<vi>)
  n195 = while {
    tunnel: w16 -> [w387]
    tunnel: w17 -> [_]
    shift-right: [w381] -> _
    shift-left: enum16{"氨氮", "总磷"}."氨氮" ("枚举") -> [w382]
    stop <- FALSE stop-if-true
    w380 = u16 3 items=["总磷"=1, "氨氮"=3] ("站号")
    # "试剂填充 172 \n管路清洗108\n氨氮92\n总磷131\n总磷海水147\n总氮76\n总氮海水92"
    n196 = Wait (ms)(milliseconds to wait=u32 1000 ("等待时间（毫秒）")) -> ()  [unwired: 1 out]
    n197 = global read "VAR氨氮全局变量.vi" "状态告警区"() -> (w378:T4)
    n198 = global read "氨氮断电保存全局变量.vi" "流程文件路径"() -> (w369:path)
    n199 = Bundle By Name(cluster=cluster{"命令":string, "data":variant} {"命令"="", "data"=variant} ("元素"), "命令"="读状态告警区", "data"=w380) -> (w389:cluster{"命令":string, "data":variant})
    n200 = local write "流程文件路径"(w369) -> ()
    n201 = Bundle By Name(cluster=cluster{"命令":string, "data":variant} {"命令"="", "data"=variant} ("元素"), "命令"="读测量数据区", "data"=w380) -> (w385:cluster{"命令":string, "data":variant})
    n202 = Unbundle By Name(w378) -> ("系统时间"=w377:timestamp)
    n203 = Enqueue Element(queue=w387, element=w389) -> (queue out=w383:refnum<queue>)  [unwired: 2 in, 2 out]
    n204 = Enqueue Element(queue=w383, element=w385) -> (queue out=w379:refnum<queue>)  [unwired: 2 in, 2 out]
    n205 = Get Date/Time In Seconds() -> (seconds since 1Jan1904=w376:timestamp)
    n206 = Subtract(x=w376, y=w377) -> (x-y=w375:dbl)
    n207 = Absolute Value(x=w375) -> (abs(x)=w374:dbl)
    n208 = global read "VAR氨氮全局变量.vi" "通讯状态"() -> (w370:bool)
    n209 = Greater Or Equal?(x=w374, y=120.0) -> (x >= y?=w372:bool)
    n210 = And(x=w370, y=w372) -> (x .and. y?=w371:bool)
    n211 = case shown="真" w371 {
      tunnel: w379 -> [_ w394]
      frame False {
      }
      frame True {
        n212 = call "氨氮启动命令.vi"("参数"=T19 {"站号"=3, "量程切换"=enum."AUTO", "控制命令"=enum."校时", "模式设置"=enum."待机", "测量间隔"=0}) -> ("启动命令"=w393:cluster{"命令":string, "data":variant})  [unwired: 10 in]
        n213 = Enqueue Element(queue=w394, element=w393) -> ()  [unwired: 2 in, 3 out]
      }
    }
    n214 = Increment(x=w382) -> (x+1=w381:enum16{"氨氮", "总磷"})
  }
  n215 = while {
    tunnel: w16 -> [w402]
    tunnel: w14 -> [w401]
    tunnel: w13 -> [w400]
    tunnel: w12 -> [w399]
    tunnel: w11 -> [w398]
    tunnel: w1 -> [w397]
    tunnel: w4 -> [w396]
    tunnel: w3 -> [_]
    stop <- FALSE stop-if-true
    n216 = event shown="[8] \"手动启动\": 值改变" {
      selector: _ -> [_ _ _ _ _ _ _ _ _ _ _ _ _ _ _ _ _ _ _]
      dyn-events: _ -> [_ _ _ _ _ _ _ _ _ _ _ _ _ _ _ _ _ _ _]
      timeout: _ -> [_ _ _ _ _ _ _ _ _ _ _ _ _ _ _ _ _ _ _]
      tunnel: w402 -> [_ w410 w439 _ _ _ _ _ w505 _ w530 w535 _ _ _ _ _ _ _]
      tunnel: w401 -> [_ _ _ _ _ _ _ _ _ _ _ _ _ _ _ w551 _ _ _]
      tunnel: w400 -> [_ _ _ _ _ _ _ _ _ _ _ _ _ _ _ w549 _ w567 w574]
      tunnel: w399 -> [_ _ _ _ _ _ _ _ _ _ _ _ _ _ _ w550 _ _ _]
      tunnel: w398 -> [_ _ _ _ _ _ _ _ _ _ _ _ _ _ _ w545 _ _ _]
      tunnel: w397 -> [_ _ _ _ _ _ _ _ _ _ _ _ _ _ _ _ _ w565 _]
      tunnel: w396 -> [_ _ _ _ _ _ _ _ _ _ _ w533 _ _ _ _ _ _ _]
      event Timeout {
        n217 = event-data() -> ()  [unwired: 1 in, 3 out]
      }
      event "串口设置": Value Change {
        n218 = event-data() -> ()  [unwired: 1 in, 6 out]
        n219 = global read "氨氮断电保存全局变量.vi" "MB通信方式选择"() -> (w404:enum16{"串口", "TCP"})
        n220 = global read "氨氮断电保存全局变量.vi" "VISA Resource"() -> (w413:refnum<visa-resource-name>)
        n221 = global read "氨氮断电保存全局变量.vi" "PORT"() -> (w408:string)
        n222 = global read "氨氮断电保存全局变量.vi" "IP"() -> (w409:string)
        n223 = call "串口配置.vi"("PORT"=w408, "IP"=w409, "MB通信方式选择"=w404, "请选择串口:"=w413) -> ("PORT 2"=w406:string, "IP 2"=w407:string, "确认 2"=w412:bool, "VISA资源名称 2"=w411:refnum<visa-resource-name>, "MB通信方式选择 2"=w405:enum16{"串口", "TCP"})  [unwired: 3 in]
        n224 = case shown="真" w412 {
          tunnel: w411 -> [_ w418]
          tunnel: w410 -> [_ w417]
          tunnel: w407 -> [_ w416]
          tunnel: w406 -> [_ w415]
          tunnel: w405 -> [_ w414]
          frame False {
          }
          frame True {
            n225 = flat-sequence {
              tunnel: w418 -> [w424]
              tunnel: w417 -> [w422]
              tunnel: w416 -> [w421]
              tunnel: w415 -> [w420]
              tunnel: w414 -> [w419]
              frame #0 {
                n226 = global write "氨氮断电保存全局变量.vi" "IP"(w421) -> ()
                n227 = global write "氨氮断电保存全局变量.vi" "PORT"(w420) -> ()
                n228 = global write "氨氮断电保存全局变量.vi" "VISA Resource"(w424) -> ()
                n229 = global write "氨氮断电保存全局变量.vi" "MB通信方式选择"(w419) -> ()
                n230 = Enqueue Element(queue=w422, element=cluster{"命令":string, "data":variant} {"命令"="启用模块", "data"=variant} ("元素")) -> ()  [unwired: 2 in, 3 out]
              }
              frame #1 {
                n231 = call <vilib>:"Application Directory.vi"() -> ("Application Directory"=w438:path)
                n232 = Build Path(base path=w438, name or relative path="data\\sys.ini" ("名称或相对路径")) -> (appended path=w436:path)
                n233 = call <vilib>:"Open Config Data.vi"("configuration file path"=w436) -> ("error out"=w432:errorcluster, "refnum"=w435:T13)  [unwired: 8 in, 1 out]
                n234 = vi-ref "氨氮断电保存全局变量.vi"() -> (w434:refnum<vi>)
                n235 = call <userlib>:"Write Panel to INI__ogtk.vi"("error in (no error)"=w432, "VI ref"=w434, "refnum"=w435) -> ("error out"=w431:errorcluster, "refnum out"=w433:T13)  [unwired: 7 in]
                n236 = call <vilib>:"Close Config Data.vi"("error in (no error)"=w431, "refnum"=w433) -> ("error out"=w426:errorcluster, "file path"=w425:path)  [unwired: 8 in]
                n237 = Open/Create/Replace File(file path (use dialog)=w425, error in=w426) -> (refnum out=w429:refnum<file>, error out=w430:errorcluster)  [unwired: 4 in, 1 out]
                n238 = Flush File(refnum=w429, error in=w430) -> (refnum out=w428:refnum<file>, error out=w427:errorcluster)
                n239 = Close File(refnum=w428, error in=w427) -> ()  [unwired: 2 out]
              }
            }
          }
        }
      }
      event "模块启用": Value Change {
        n240 = event-data() -> ("OldVal"=w440:bool)  [unwired: 1 in, 5 out]
        n241 = case shown="假" w440 {
          tunnel: w439 -> [w441 w443]
          frame False {
            n242 = Enqueue Element(queue=w441, element=cluster{"命令":string, "data":variant} {"命令"="停用模块", "data"=variant} ("元素")) -> ()  [unwired: 2 in, 3 out]
          }
          frame True {
            n243 = Enqueue Element(queue=w443, element=cluster{"命令":string, "data":variant} {"命令"="启用模块", "data"=variant} ("元素")) -> ()  [unwired: 2 in, 3 out]
          }
        }
      }
      event "流程文件路径": Value Change {
        n244 = event-data() -> ()  [unwired: 1 in, 6 out]
        n245 = flat-sequence {
          frame #0 {
            n246 = local read "流程文件路径"() -> (w445:path)
            n247 = global write "氨氮断电保存全局变量.vi" "流程文件路径"(w445) -> ()
          }
          frame #1 {
            n248 = call <vilib>:"Application Directory.vi"() -> ("Application Directory"=w459:path)
            n249 = Build Path(base path=w459, name or relative path="data\\sys.ini" ("名称或相对路径")) -> (appended path=w457:path)
            n250 = call <vilib>:"Open Config Data.vi"("configuration file path"=w457) -> ("error out"=w453:errorcluster, "refnum"=w456:T13)  [unwired: 8 in, 1 out]
            n251 = vi-ref "氨氮断电保存全局变量.vi"() -> (w455:refnum<vi>)
            n252 = call <userlib>:"Write Panel to INI__ogtk.vi"("error in (no error)"=w453, "VI ref"=w455, "refnum"=w456) -> ("error out"=w452:errorcluster, "refnum out"=w454:T13)  [unwired: 7 in]
            n253 = call <vilib>:"Close Config Data.vi"("error in (no error)"=w452, "refnum"=w454) -> ("error out"=w447:errorcluster, "file path"=w446:path)  [unwired: 8 in]
            n254 = Open/Create/Replace File(file path (use dialog)=w446, error in=w447) -> (refnum out=w450:refnum<file>, error out=w451:errorcluster)  [unwired: 4 in, 1 out]
            n255 = Flush File(refnum=w450, error in=w451) -> (refnum out=w449:refnum<file>, error out=w448:errorcluster)
            n256 = Close File(refnum=w449, error in=w448) -> ()  [unwired: 2 out]
          }
        }
      }
      event "公式一键写入": Value Change {
        n257 = event-data() -> ()  [unwired: 1 in, 6 out]
        n258 = local read "公式"() -> (w460:cluster{"X^2":dbl, "X":dbl, "b":dbl})
        n259 = call "公式复合写入.vi"("公式"=w460) -> ()  [unwired: 11 in]
      }
      event "曲线模型": Value Change {
        n260 = event-data() -> ()  [unwired: 1 in, 6 out]
        n261 = local write "公式"("曲线模型") -> ()
      }
      event "质控参数设置": Value Change {
        n262 = event-data() -> ()  [unwired: 1 in, 6 out]
        n263 = global read "氨氮断电保存全局变量.vi" "质控参数设置"() -> (w462:T20)
        n264 = call "质控参数设置.vi"("质控参数设置"=w462) -> ("输出簇"=w463:T21)  [unwired: 10 in]
        n265 = Unbundle By Name(w463) -> ("确定"=w464:bool)
        n266 = case shown="真" w464 {
          tunnel: w463 -> [_ w466]
          tunnel: w462 -> [_ w465]
          frame False {
          }
          frame True {
            n267 = flat-sequence {
              tunnel: w466 -> [w473]
              tunnel: w465 -> [w467]
              frame #0 {
                n268 = Unbundle By Name(w473) -> ("跨度值"=w472:dbl, "零点标准液浓度"=w471:dbl, "跨度标准液浓度"=w470:dbl, "标准液标准浓度"=w469:dbl)
                n269 = Bundle By Name(cluster=w467, "跨度值"=w472, "零点标准液浓度"=w471, "跨度标准液浓度"=w470, "标准液标准浓度"=w469) -> (w468:T20)
                n270 = global write "氨氮断电保存全局变量.vi" "质控参数设置"(w468) -> ()
              }
              frame #1 {
                n271 = call <vilib>:"Application Directory.vi"() -> ("Application Directory"=w474:path)
                n272 = Build Path(base path=w474, name or relative path="data\\sys.ini" ("名称或相对路径")) -> (appended path=w476:path)
                n273 = call <vilib>:"Open Config Data.vi"("configuration file path"=w476) -> ("error out"=w480:errorcluster, "refnum"=w477:T13)  [unwired: 8 in, 1 out]
                n274 = vi-ref "氨氮断电保存全局变量.vi"() -> (w478:refnum<vi>)
                n275 = call <userlib>:"Write Panel to INI__ogtk.vi"("error in (no error)"=w480, "VI ref"=w478, "refnum"=w477) -> ("error out"=w481:errorcluster, "refnum out"=w479:T13)  [unwired: 7 in]
                n276 = call <vilib>:"Close Config Data.vi"("error in (no error)"=w481, "refnum"=w479) -> ("error out"=w486:errorcluster, "file path"=w487:path)  [unwired: 8 in]
                n277 = Open/Create/Replace File(file path (use dialog)=w487, error in=w486) -> (refnum out=w483:refnum<file>, error out=w482:errorcluster)  [unwired: 4 in, 1 out]
                n278 = Flush File(refnum=w483, error in=w482) -> (refnum out=w484:refnum<file>, error out=w485:errorcluster)
                n279 = Close File(refnum=w484, error in=w485) -> ()  [unwired: 2 out]
              }
            }
          }
        }
      }
      event "氨氮自动测试量程配置": Value Change {
        n280 = event-data() -> ()  [unwired: 1 in, 6 out]
        n281 = flat-sequence {
          frame #0 {
            n282 = global write "氨氮断电保存全局变量.vi" "氨氮自动测试量程配置"("氨氮自动测试量程配置") -> ()
          }
          frame #1 {
            n283 = call <vilib>:"Application Directory.vi"() -> ("Application Directory"=w502:path)
            n284 = Build Path(base path=w502, name or relative path="data\\sys.ini" ("名称或相对路径")) -> (appended path=w500:path)
            n285 = call <vilib>:"Open Config Data.vi"("configuration file path"=w500) -> ("error out"=w496:errorcluster, "refnum"=w499:T13)  [unwired: 8 in, 1 out]
            n286 = vi-ref "氨氮断电保存全局变量.vi"() -> (w498:refnum<vi>)
            n287 = call <userlib>:"Write Panel to INI__ogtk.vi"("error in (no error)"=w496, "VI ref"=w498, "refnum"=w499) -> ("error out"=w495:errorcluster, "refnum out"=w497:T13)  [unwired: 7 in]
            n288 = call <vilib>:"Close Config Data.vi"("error in (no error)"=w495, "refnum"=w497) -> ("error out"=w490:errorcluster, "file path"=w489:path)  [unwired: 8 in]
            n289 = Open/Create/Replace File(file path (use dialog)=w489, error in=w490) -> (refnum out=w493:refnum<file>, error out=w494:errorcluster)  [unwired: 4 in, 1 out]
            n290 = Flush File(refnum=w493, error in=w494) -> (refnum out=w492:refnum<file>, error out=w491:errorcluster)
            n291 = Close File(refnum=w492, error in=w491) -> ()  [unwired: 2 out]
          }
        }
      }
      event "手动启动": Value Change {
        n292 = event-data() -> ()  [unwired: 1 in, 6 out]
        n293 = call "氨氮启动参数对话框.vi"() -> ("确认"=w503:bool, "元素"=w504:cluster{"命令":string, "data":variant})  [unwired: 10 in]
        n294 = case shown="真" w503 {
          tunnel: w505 -> [_ w507]
          tunnel: w504 -> [_ w506]
          frame False {
          }
          frame True {
            n295 = Enqueue Element(queue=w507, element=w506) -> ()  [unwired: 2 in, 3 out]
          }
        }
      }
      event "定时启动": Mouse Down {
        n296 = event-data() -> ()  [unwired: 1 in, 6 out]
        n297 = flat-sequence {
          frame #0 {
            n298 = global read "氨氮断电保存全局变量.vi" "定时控制"() -> (w508:T6)
            n299 = call "周期设置.vi"("定时控制输入"=w508) -> ("定时控制输出"=w509:T22)  [unwired: 10 in]
            n300 = global write "氨氮断电保存全局变量.vi" "定时控制"(w509) -> ()
          }
          frame #1 {
            n301 = call <vilib>:"Application Directory.vi"() -> ("Application Directory"=w523:path)
            n302 = Build Path(base path=w523, name or relative path="data\\sys.ini" ("名称或相对路径")) -> (appended path=w521:path)
            n303 = call <vilib>:"Open Config Data.vi"("configuration file path"=w521) -> ("error out"=w517:errorcluster, "refnum"=w520:T13)  [unwired: 8 in, 1 out]
            n304 = vi-ref "氨氮断电保存全局变量.vi"() -> (w519:refnum<vi>)
            n305 = call <userlib>:"Write Panel to INI__ogtk.vi"("error in (no error)"=w517, "VI ref"=w519, "refnum"=w520) -> ("error out"=w516:errorcluster, "refnum out"=w518:T13)  [unwired: 7 in]
            n306 = call <vilib>:"Close Config Data.vi"("error in (no error)"=w516, "refnum"=w518) -> ("error out"=w511:errorcluster, "file path"=w510:path)  [unwired: 8 in]
            n307 = Open/Create/Replace File(file path (use dialog)=w510, error in=w511) -> (refnum out=w514:refnum<file>, error out=w515:errorcluster)  [unwired: 4 in, 1 out]
            n308 = Flush File(refnum=w514, error in=w515) -> (refnum out=w513:refnum<file>, error out=w512:errorcluster)
            n309 = Close File(refnum=w513, error in=w512) -> ()  [unwired: 2 out]
          }
        }
      }
      event "单步测试": Value Change {
        w525 = u16 1 items=["总磷"=1, "氨氮"=3] ("站号")
        n310 = event-data() -> ()  [unwired: 1 in, 6 out]
        n311 = Bundle("站号"=w525, "总磷氨氮调试"="总磷氨氮调试") -> (w524:cluster{"站号":u16, "总磷氨氮调试":u16[]})  [unwired: 1 in]
        n312 = Bundle By Name(cluster=cluster{"命令":string, "data":variant} {"命令"="", "data"=variant} ("元素"), "命令"="debug", "data"=w524) -> (w527:cluster{"命令":string, "data":variant})
        n313 = Enqueue Element(queue=w530, element=w527) -> ()  [unwired: 2 in, 3 out]
      }
      event "停止": Value Change {
        n314 = event-data() -> ()  [unwired: 1 in, 6 out]
        n315 = Enqueue Element(queue=w535, element=cluster{"命令":string, "data":variant} {"命令"="启动", "data"=variant(cluster{"站号":u16, "控制命令输出":u16[]} {"站号"=3, "控制命令输出"=[2816]})} ("启动命令")) -> ()  [unwired: 2 in, 3 out]
        n316 = Cancel Notification(0:w533) -> (8:w532:refnum<notifier>)  [unwired: 1 in, 2 out]
        n317 = Send Notification(notification=TRUE ("通知"), notifier=w532) -> ()  [unwired: 1 in, 2 out]
      }
      event "设置": Value Change {
        n318 = event-data() -> ()  [unwired: 1 in, 6 out]
        n319 = property on="窗格" class="Pane"("Origin"=T10 {"Horizontal"=0, "Vertical"=628} ("原点")) -> ()  [unwired: 2 in, 2 out]
      }
      event "返回": Value Change {
        n320 = event-data() -> ()  [unwired: 1 in, 6 out]
        n321 = property on="窗格" class="Pane"("Origin"=T10 {"Horizontal"=0, "Vertical"=0} ("原点")) -> ()  [unwired: 2 in, 2 out]
      }
      event "公式.X^2", "公式.X", "公式.b": Mouse Down {
        n322 = event-data() -> ("CtlRef"=w541:refnum<vi>)  [unwired: 1 in, 5 out]
        n323 = property class="DigNum (严格)"(reference=w541) -> (reference out=w539:refnum<vi>, "Value"=w540:dbl)  [unwired: 1 in, 1 out]
        n324 = call "数字键盘.vi"("OldNumber"=w540) -> ("NewNumber"=w538:dbl)
        n325 = property class="DigNum (严格)"(reference=w539, "Val(Sgnl)"=w538) -> ()  [unwired: 1 in, 2 out]
      }
      event "读公式": Value Change {
        n326 = event-data() -> ()  [unwired: 1 in, 6 out]
        n327 = property class="Enum (严格)"(reference=w549) -> ("Value"=w548:enum16{"氨氮", "总磷"})  [unwired: 1 in, 2 out]
        n328 = property class="Enum (严格)"(reference=w550) -> ("Value"=w547:enum16{"水样测量", "空白核查", "跨度核查", "标样核查", "加标回收"})  [unwired: 1 in, 2 out]
        n329 = property class="Enum (严格)"(reference=w551) -> ("Value"=w546:enum16{"低量程", "高量程"})  [unwired: 1 in, 2 out]
        n330 = call "总磷氨氮公式读取_N.vi"("量程"=w546, "测量模式"=w547, "测量参数"=w548) -> ("error out"=w543:errorcluster, "公式"=w544:cluster{"X^2":dbl, "X":dbl, "b":dbl})  [unwired: 7 in]
        n331 = property class="Clust (严格)"(reference=w545, "Value"=w544) -> ()  [unwired: 1 in, 2 out]
        n332 = case shown="错误" w543 {
          tunnel: ["读取成功" ("消息") "读取失败" ("消息")] -> w542
          frame No Error {
          }
          frame Error {
          }
        }
        n333 = One Button Dialog(message=w542) -> ()  [unwired: 1 in, 1 out]
      }
      event "写公式": Value Change {
        n334 = event-data() -> ()  [unwired: 1 in, 6 out]
        n335 = call "总磷氨氮公式写入_N.vi"("公式"="公式", "量程"="量程下拉列表", "测量模式"="测量模式下拉列表", "测量参数"="参数下拉列表") -> ("error out"=w554:errorcluster)  [unwired: 7 in]
        n336 = case shown="无错误" w554 {
          tunnel: ["写入成功" ("消息") "写入失败" ("消息")] -> w555
          frame No Error {
          }
          frame Error {
          }
        }
        n337 = One Button Dialog(message=w555) -> ()  [unwired: 1 in, 1 out]
      }
      event "备用系数读取": Value Change {
        n338 = event-data() -> ()  [unwired: 1 in, 6 out]
        n339 = property class="Enum (严格)"(reference=w567) -> ("Value"=w566:enum16{"氨氮", "总磷"})  [unwired: 1 in, 2 out]
        n340 = call "总磷氨氮量程读取N.vi"("测量参数"=w566) -> ("error out"=w563:errorcluster, "量程参数读取"=w562:T1)  [unwired: 9 in]
        n341 = property class="Clust (严格)"(reference=w565, "Value"=w562) -> ()  [unwired: 1 in, 2 out]
        n342 = case shown="错误" w563 {
          tunnel: ["读取成功" ("消息") "读取失败" ("消息")] -> w564
          frame No Error {
          }
          frame Error {
          }
        }
        n343 = One Button Dialog(message=w564) -> ()  [unwired: 1 in, 1 out]
      }
      event "备用系数写入": Value Change {
        n344 = event-data() -> ()  [unwired: 1 in, 6 out]
        n345 = property class="Enum (严格)"(reference=w574) -> ("Value"=w573:enum16{"氨氮", "总磷"})  [unwired: 1 in, 2 out]
        n346 = call "总磷氨氮量程写入N.vi"("量程参数写入"="量程参数读取", "测量参数"=w573) -> ("error out"=w571:errorcluster)  [unwired: 8 in]
        n347 = case shown="无错误" w571 {
          tunnel: ["写入成功" ("消息") "写入失败" ("消息")] -> w572
          frame No Error {
          }
          frame Error {
          }
        }
        n348 = One Button Dialog(message=w572) -> ()  [unwired: 1 in, 1 out]
      }
    }
  }
